vi "xPCGetParamIdx.vi"(3 "error in (no error)":errorcluster, 4 "blockpath":string, 5 "parametername":string, 6 "port":i32) -> (0 "error out":errorcluster, 1 "identifier":i32, 2 "port copy":i32)   [LabVIEW 2018]
uses:
  xpcapi.dll
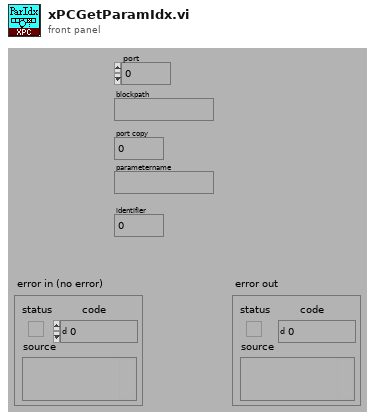
[diagram p1: front panel]
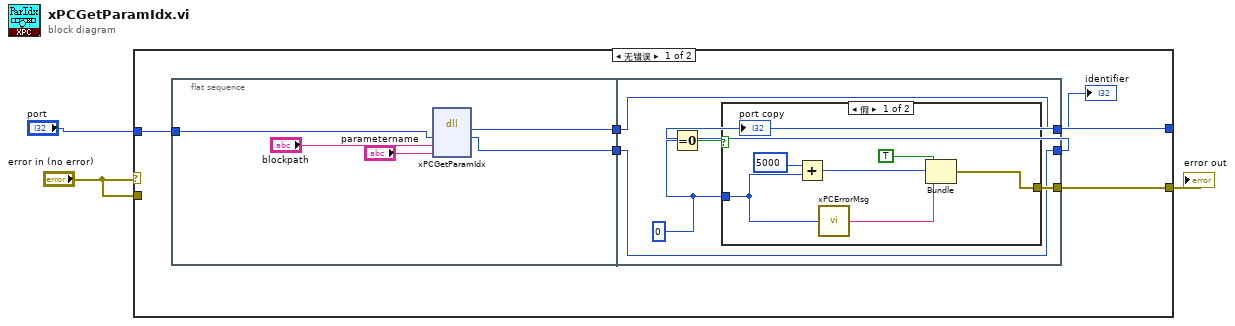
[diagram p0: block diagram]
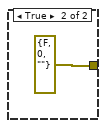
[diagram p2: hidden frame]
diagram:
  n1 = case shown="无错误" "error in (no error)" {
    tunnel: [w10 w29] -> w4
    tunnel: "error in (no error)" -> [_ w29]
    tunnel: "port" -> [w8 w28]
    tunnel: [w9 w28] -> w2
    frame No Error {
      n2 = flat-sequence {
        tunnel: [w12] -> w6
        tunnel: w8 -> [w13]
        tunnel: [w11] -> w5
        tunnel: [w18] -> w9
        tunnel: w6 -> [w18]
        tunnel: [w19] -> w10
        tunnel: [w17] -> w7
        tunnel: w5 -> [w17]
        frame #0 {
          n3 = dll-call lib="PTH2;abs CUsers\nAdministratorDesktop备份3\nxpcapi.dll" fn="xPCGetParamIdx"("port"=w13, "blockpath"="blockpath", "parametername"="parametername") -> (w11:i32, "port"=w12:i32)  [unwired: 5 in, 2 out]
        }
        frame #1 {
          w16 = 0
          n4 = Equal To 0?(x=w16) -> (x = 0?=w20:bool)
          n5 = case shown="假" w20 {
            tunnel: w16 -> [w22 _]
            tunnel: [w23 errorcluster {"status"=FALSE, "code"=0, "source"=""} ("error out")] -> w19
            frame False {
              n6 = Add(x=5000 ("y"), y=w22) -> (x+y=w25:i32)
              n7 = call "xPCErrorMsg.vi"("error number"=w22) -> ("ErrorMsg"=w24:string)
              n8 = Bundle(TRUE, w25, "ErrorMsg"=w24) -> (w23:cluster{bool, i32, "ErrorMsg":string})  [unwired: 1 in]
            }
            frame True {
            }
          }
        }
      }
      "identifier" <- w7
    }
    frame Error {
    }
  }
  "port copy" <- w2
  "error out" <- w4
